vi "Webcam Optical Flow.vi"() -> ()   [LabVIEW 2014]
uses:
  <vilib>/userdefined/High Color/IMAQdx.ctl
  <vilib>/vision/driver/NI_Vision_Acquisition_Software.lvlib
  <vilib>/vision/NI_Vision_Development_Module.lvlib
panel:
  in  "Set ROI":bool
  out "x-y":u32
  out "appended array":sgl[](array[numeric])
  in  "disabled index (col)":i32
  in  "index (row)":i32
  in  "Window Size (15x15)":cluster{"Size X":i32, "Size Y":i32}={"Size X"=15, "Size Y"=15}
  out "error out 2":errorcluster
  in  "Stop":bool
  out "Image":T1(plugin-control)
  out "error out":errorcluster
  in  "Session In":T2="cam0"
  # "Pixel Coordinates"
  # "Velocity of the pixel (Vx, Vy)"
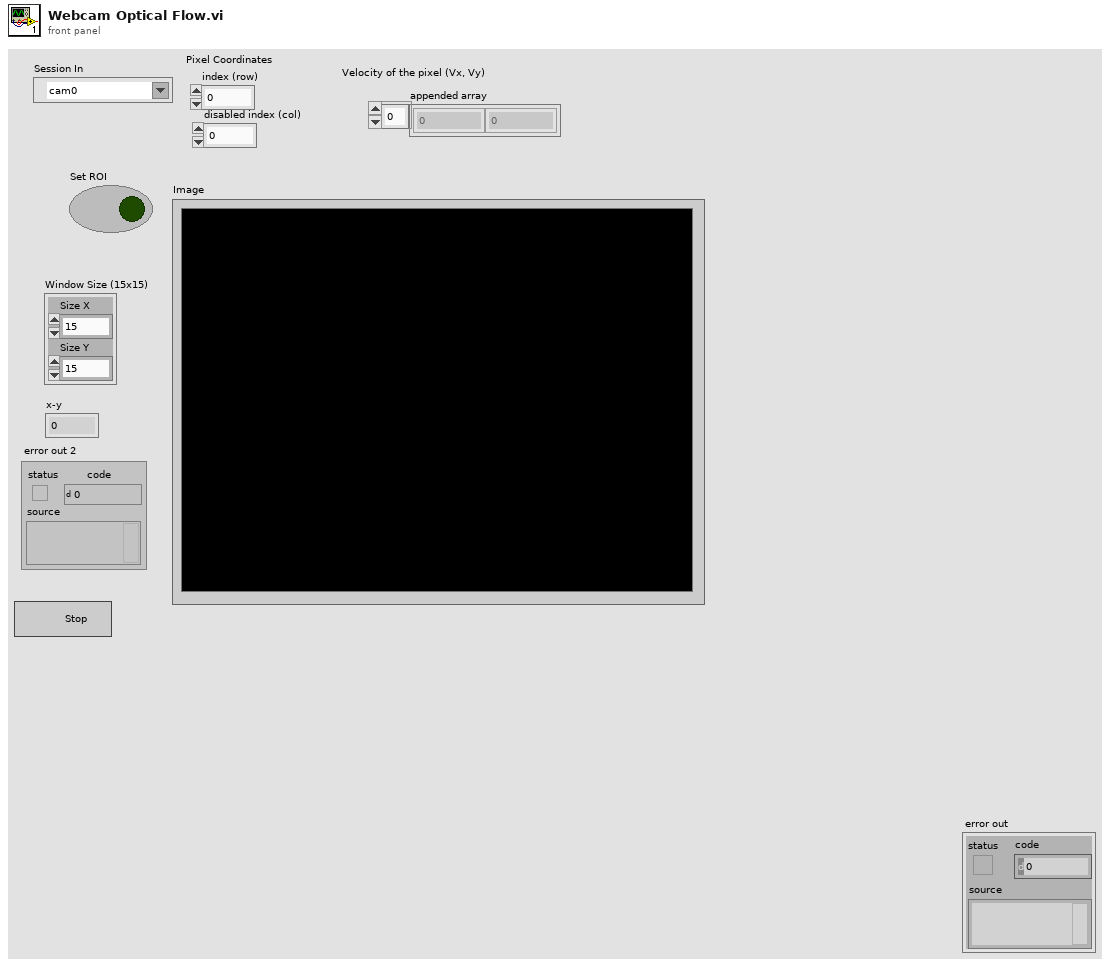
[diagram p1: front panel]
types:
  T1 = typedef "IMAQ Image.ctl" = refnum<image>
  T2 = typedef "IMAQdx.ctl" = refnum<k21>
  T3 = typedef "Image Type" = u32
  T4 = typedef "IMAQ Rectangle" = cluster{"Left":i32, "Top":i32, "Right":i32, "Bottom":i32, "Rotation":dbl}
  T5 = typedef "ROI Descriptor" = cluster{"Global Rectangle":i32[], "Contours":cluster{"ID":enum32{"External", "Internal"}, "Type":u32, "Coordinates":i32[]}[]}
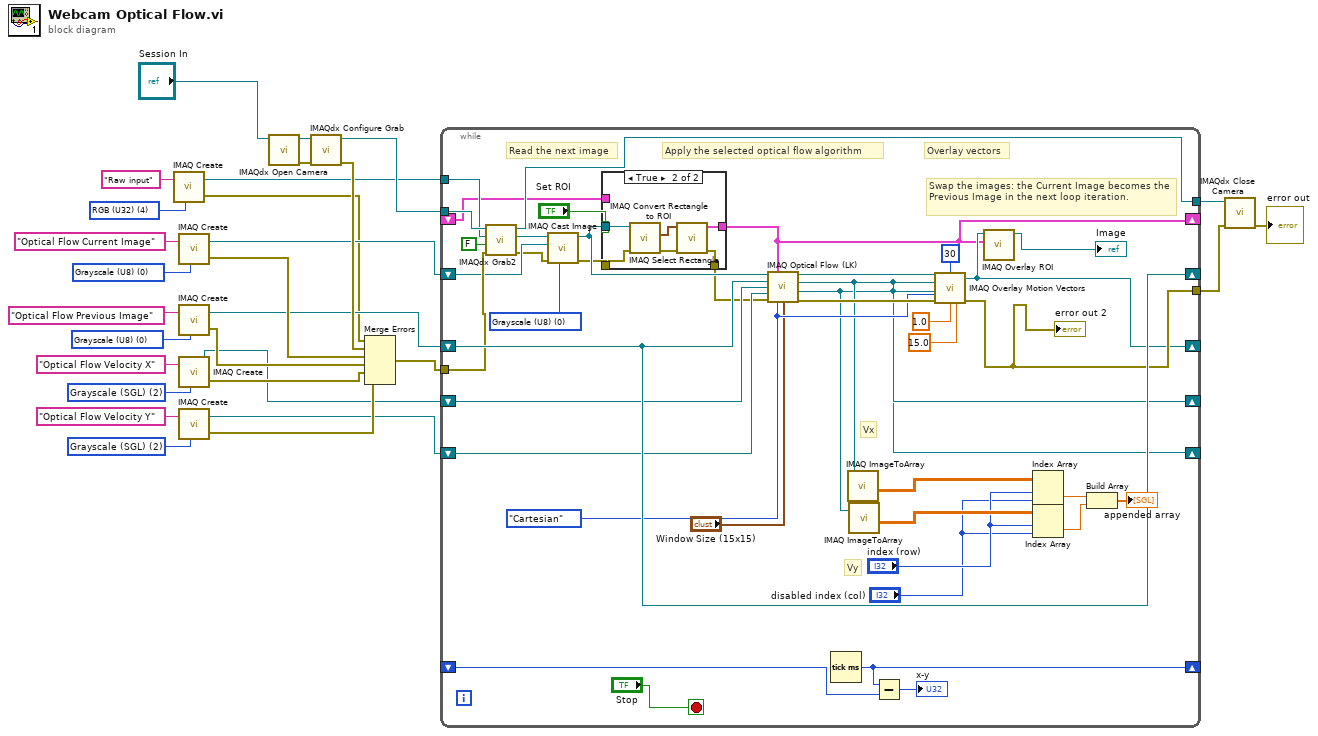
[diagram p0: block diagram]
diagram:
  w3 = T3 4 items=["Grayscale (U8)", "Grayscale (I16)", "Grayscale (SGL)", "Complex (CSG)", "RGB (U32)", "HSL (U32)", "RGB (U64)", "Grayscale (U16)"] ("Image Type")
  w19 = T3 2 items=["Grayscale (U8)", "Grayscale (I16)", "Grayscale (SGL)", "Complex (CSG)", "RGB (U32)", "HSL (U32)", "RGB (U64)", "Grayscale (U16)"] ("Image Type")
  w20 = T3 0 items=["Grayscale (U8)", "Grayscale (I16)", "Grayscale (SGL)", "Complex (CSG)", "RGB (U32)", "HSL (U32)", "RGB (U64)", "Grayscale (U16)"] ("Image Type")
  w21 = T3 0 items=["Grayscale (U8)", "Grayscale (I16)", "Grayscale (SGL)", "Complex (CSG)", "RGB (U32)", "HSL (U32)", "RGB (U64)", "Grayscale (U16)"] ("Image Type")
  w22 = T3 2 items=["Grayscale (U8)", "Grayscale (I16)", "Grayscale (SGL)", "Complex (CSG)", "RGB (U32)", "HSL (U32)", "RGB (U64)", "Grayscale (U16)"] ("Image Type")
  n1 = call "IMAQ Create"("Image Name"="Raw input", "Image Type"=w3) -> ("New Image"=w1:T1, "error out"=w2:errorcluster)  [unwired: 2 in, 1 out]
  n2 = call "IMAQ Create"("Image Name"="Optical Flow Current Image", "Image Type"=w21) -> ("New Image"=w11:T1, "error out"=w16:errorcluster)  [unwired: 2 in, 1 out]
  n3 = call "IMAQ Create"("Image Name"="Optical Flow Previous Image", "Image Type"=w20) -> ("New Image"=w9:T1, "error out"=w15:errorcluster)  [unwired: 2 in, 1 out]
  n4 = call "IMAQ Create"("Image Name"="Optical Flow Velocity X", "Image Type"=w22) -> ("New Image"=w8:T1, "error out"=w14:errorcluster)  [unwired: 2 in, 1 out]
  n5 = call "IMAQ Create"("Image Name"="Optical Flow Velocity Y", "Image Type"=w19) -> ("New Image"=w7:T1, "error out"=w13:errorcluster)  [unwired: 2 in, 1 out]
  n6 = call <vilib>:"IMAQdx Open Camera.vi"("Session In"="Session In") -> ("error out"=w28:errorcluster, "Session Out"=w29:T2)  [unwired: 9 in]
  n7 = call <vilib>:"IMAQdx Configure Grab.vi"("error in"=w28, "Session In"=w29) -> ("error out"=w17:errorcluster, "Session Out"=w12:T2)  [unwired: 8 in]
  n8 = Merge Errors(w2, w17, w16, w15, w14, w13) -> (w10:errorcluster)
  n9 = while {
    tunnel: [w53] -> w5
    shift-right: [w50] -> _
    shift-left: w8 -> [w69]
    shift-right: [w49] -> _
    shift-left: w7 -> [w68]
    shift-right: [w34] -> _
    shift-left: w9 -> [w70]
    tunnel: w10 -> [w61]
    shift-right: [w70] -> _
    shift-left: w11 -> [w57]
    tunnel: w12 -> [w62]
    tunnel: [w59] -> w6
    tunnel: w1 -> [w54]
    shift-right: [w41] -> _
    shift-left: _ -> [w40]
    shift-right: [w32] -> _
    shift-left: _ -> [w31]
    stop <- "Stop" stop-if-true
    w55 = T3 0 items=["Grayscale (U8)", "Grayscale (I16)", "Grayscale (SGL)", "Complex (CSG)", "RGB (U32)", "HSL (U32)", "RGB (U64)", "Grayscale (U16)"] ("Image Type")
    w52 = enum16{"Cartesian", "Polar"}."Cartesian" ("Velocity Representation")
    # "Vy"
    # "Vx"
    # "Swap the images: the Current Image becomes the Previous Image in the next loop iteration."
    # "Overlay vectors"
    # "Read the next image"
    # "Apply the selected optical flow algorithm"
    n10 = call <vilib>:"IMAQdx Grab2.vi"("error in"=w61, "Wait for Next Buffer? (Yes)"=FALSE, "Image In"=w54, "Session In"=w62) -> ("error out"=w56:errorcluster, "Image Out"=w58:T1, "Session Out"=w59:T2)  [unwired: 4 in, 1 out]
    n11 = call "IMAQ Cast Image"("Image Type"=w55, "error in (no error)"=w56, "Image Dst"=w57, "Image Src"=w58) -> ("error out"=w37:errorcluster, "Image Dst Out"=w38:T1)  [unwired: 6 in]
    n12 = case shown="True" "Set ROI" {
      tunnel: w38 -> [_ w78]
      tunnel: [w71 w76] -> w32
      tunnel: w37 -> [w72 w75]
      tunnel: [w72 w74] -> w36
      tunnel: w31 -> [w71 _]
      frame False {
      }
      frame True {
        n13 = call "IMAQ Select Rectangle"("error in (no error)"=w75, "Image In"=w78) -> ("error out"=w77:errorcluster, "Rectangle"=w73:T4)  [unwired: 6 in, 2 out]
        n14 = call "IMAQ Convert Rectangle to ROI"("error in (no error)"=w77, "Rectangle"=w73) -> ("error out"=w74:errorcluster, "ROI Descriptor"=w76:T5)  [unwired: 7 in]
      }
    }
    n15 = call "IMAQ Optical Flow (LK)"("Current Frame"=w38, "ROI Descriptor"=w32, "Previous Frame"=w70, "Velocity Component 1 In"=w69, "Velocity Component 2 In"=w68, "error in (no error)"=w36, "Velocity Representation"=w52, "Window Size (15x15)"="Window Size (15x15)") -> ("Current Frame Out (dup)"=w66:T1, "Velocity Component 1 Out"=w50:T1, "Velocity Component 2 Out"=w49:T1, "error out"=w67:errorcluster)  [unwired: 4 out]
    n16 = Tick Count (ms)() -> (millisecond timer value=w41:u32)
    n17 = call "IMAQ ImageToArray"("Image"=w50) -> ("Image Pixels (Float)"=w48:sgl[][])  [unwired: 3 in, 4 out]
    n18 = call "IMAQ ImageToArray"("Image"=w49) -> ("Image Pixels (Float)"=w47:sgl[][])  [unwired: 3 in, 4 out]
    n19 = Subtract(x=w41, y=w40) -> (x-y=→"x-y":u32)
    n20 = call "IMAQ Overlay Motion Vectors"("Image"=w66, "Step Size"=30, "Velocity Component 1"=w50, "Velocity Component 2"=w49, "Velocity Representation"=w52, "error in (no error)"=w67, "Scale"=1.0, "Threshold"=15.0) -> ("Image Out"=w34:T1, "error out"=w53:errorcluster)  [unwired: 2 in, 4 out]
    "error out 2" <- w53
    n21 = call "IMAQ Overlay ROI"("ROI Descriptor"=w32, "Image"=w34) -> ("Image Out"=→"Image":T1)  [unwired: 8 in, 1 out]
    n22 = Index Array(array=w48, index (row)="index (row)", index (col)="disabled index (col)") -> (element=w44:sgl)
    n23 = Index Array(array=w47, index (row)="index (row)", index (col)="disabled index (col)") -> (element=w43:sgl)
    n24 = Build Array(w44, w43) -> (→"appended array":sgl[])
  }
  n25 = call <vilib>:"IMAQdx Close Camera.vi"("error in"=w5, "Session In"=w6) -> ("error out"=→"error out":errorcluster)  [unwired: 9 in]
